vi "Read Show Time.vi"(8 "error in (no error)":errorcluster, 11 "MGI_Progress Bar Options in":refnum<class "Progress Bar Settings.lvclass">) -> (0 "error out":errorcluster, 2 "Show Time":bool, 3 "MGI_Progress Bar Options out":refnum<class "Progress Bar Settings.lvclass">)   [LabVIEW 2016, in "Progress Bar Settings.lvclass"]
uses:
  <userlib>/_MGI/User Interface/Progress Bar/Progress Bar Settings/Progress Bar Settings.lvclass
  <userlib>/_MGI/User Interface/Progress Bar/Progress Bar Settings/Progress Bar Settings.lvclass/Progress Bar Settings.ctl
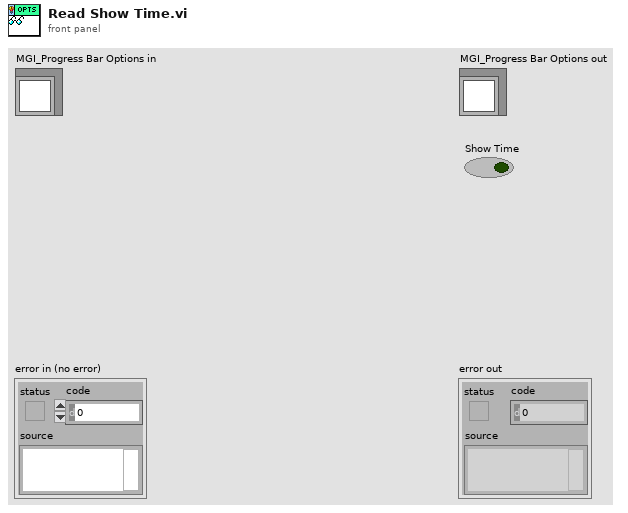
[diagram p1: front panel]
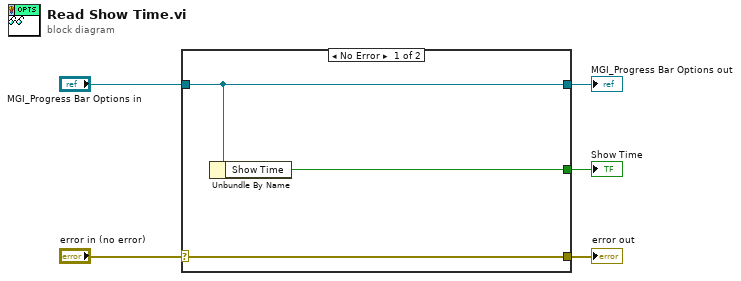
[diagram p0: block diagram]
diagram:
  n1 = case shown="No Error" "error in (no error)" {
    selector: "error in (no error)" -> [w8 w9]
    tunnel: [w8 w9] -> w4
    tunnel: [w7 w10] -> w2
    tunnel: "MGI_Progress Bar Options in" -> [w7 w10]
    tunnel: [w6 _] -> w1
    frame No Error {
      n2 = Unbundle By Name(w7) -> ("Show Time"=w6:bool)
    }
    frame Error {
    }
  }
  "error out" <- w4
  "MGI_Progress Bar Options out" <- w2
  "Show Time" <- w1
